vi "Main Tclk.vi"() -> ()   [LabVIEW 2018] (continued)
                        n7248 = Bundle By Name(cluster=w1400, "Low mag scan"=w1398, "Prior to main scan"=w1397, "Low mag interval"=w1396, "Low mag scan rate (Hz)"=w1395, "Show HM box"=w1394) -> (w1399:T30)
                        n7249 = local write "Low Mag SEM"(w1399) -> ()
                        n7250 = local write "Mid Mag SEM"(w1392) -> ()
                      }
                      frame #2 {
                        n7251 = Unbundle By Name(w1407) -> ("Line milling time (s)"=w1404:sgl, "Lines auto pause"=w1403:u16, "Auto Profile"=w1402:bool)
                        n7252 = local read "Milling para"() -> (w1406:T35)
                        n7253 = Bundle By Name(cluster=w1406, "Line milling time (s)"=w1404, "Lines auto pause"=w1403, "Auto Profile"=w1402) -> (w1405:T35)
                        n7254 = local write "Milling para"(w1405) -> ()
                      }
                    }
                  }
                  frame True {
                    n7255 = local write "SEM Scan Parameters"(w1427) -> ()
                    n7256 = local write "Detector Information"(w1413) -> ()
                    n7257 = local write "SEM Options"(w1426) -> ()
                    n7258 = local write "File Information"(w1425) -> ()
                    n7259 = local write "Low Mag SEM"(w1424) -> ()
                    n7260 = local write "Mid Mag SEM"(w1416) -> ()
                    n7261 = local write "FIB-SEM Angle"(w1423) -> ()
                    n7262 = local write "Milling para"(w1422) -> ()
                    n7263 = local write "X shift (nm/image)"(w1420) -> ()
                    n7264 = local write "Y shift (nm/image)"(w1421) -> ()
                    n7265 = local write "FIB Y zoom pixel (nm)"(w1419) -> ()
                    n7266 = local write "Mail server"(w1418) -> ()
                    n7267 = local write "Email Alert Recipients"(w1417) -> ()
                    n7268 = Unbundle By Name(w1413) -> ("Brightness A"=w1412:dbl, "Contrast A"=w1411:dbl, "Detector B name"=w1410:string, "Brightness B"=w1409:dbl, "Contrast B"=w1408:dbl)
                    n7269 = local read "Hardware Configuration"() -> (w1415:T25)
                    n7270 = Bundle By Name(cluster=w1415, "Brightness A"=w1412, "Contrast A"=w1411, "Detector B name"=w1410, "Brightness B"=w1409, "Contrast B"=w1408) -> (w1414:T25)
                    n7271 = local write "Hardware Configuration"(w1414) -> ()
                  }
                }
              }
              frame #1 {
                n7272 = local read "Hardware Configuration"() -> (w1448:T25)
                n7273 = local read "SEM Scan Parameters"() -> (w1432:T26)
                n7274 = local read "SEM Options"() -> (w1449:T27)
                n7275 = local read "SEM Status"() -> (w1450:T12)
                n7276 = local read "X full scale (V)"() -> (w1451:sgl)
                n7277 = local read "Mid Mag SEM"() -> (w1447:T29)
                n7278 = local read "SEM Mid Mag Scan Parameters"() -> (w1446:T5)
                n7279 = Unbundle By Name(w1447) -> ("X size (um)"=w1443:sgl, "Y size (um)"=w1442:sgl, "X center (um)"=w1441:dbl, "Y center (um)"=w1440:dbl, "Mid mag scan rate (Hz)"=w1445:u32, "Pixel size (nm)"=w1444:sgl)
                n7280 = call "SEM Scan Parameter Coerce.vi"("X full scale (V)"=w1451, "AI upper limit"=50000000.0, "SEM Status"=w1450, "SEM Options"=w1449, "SEM Scan Parameters"=w1432, "Hardware Configuration"=w1448) -> ("Coerced SEM Scan Parameters"=w1452:T5, "SEM FOV"=w1431:dbl, "Detector number"=w1430:i16)  [unwired: 3 in]
                n7281 = local write "Detector number"(w1430) -> ()
                n7282 = local write "SEM FOV"(w1431) -> ()
                n7283 = Bundle By Name(cluster=w1446, "X size (um)"=w1443, "Y size (um)"=w1442, "X center (um)"=w1441, "Y center (um)"=w1440, "Scan rate (Hz)"=w1445, "Pixel size (nm)"=w1444, "X size auto"=TRUE) -> (w1439:T5)
                n7284 = call "SEM Scan Parameter Coerce.vi"("X full scale (V)"=w1451, "SEM Status"=w1450, "SEM Options"=w1449, "SEM Scan Parameters"=w1439, "Hardware Configuration"=w1448) -> ("Coerced SEM Scan Parameters"=w1453:T5)  [unwired: 4 in, 2 out]
                n7285 = Unbundle By Name(w1453) -> ("X size (um)"=w1438:sgl, "Y size (um)"=w1437:sgl, "X center (um)"=w1436:dbl, "Y center (um)"=w1435:dbl, "Scan rate (Hz)"=w1434:u32, "Pixel size (nm)"=w1433:sgl)
                n7286 = Bundle By Name(cluster=w1447, "X size (um)"=w1438, "Y size (um)"=w1437, "X center (um)"=w1436, "Y center (um)"=w1435, "Mid mag scan rate (Hz)"=w1434, "Pixel size (nm)"=w1433) -> (w1454:T29)
                n7287 = local write "SEM Scan Parameters"(w1452) -> ()
                n7288 = local write "SEM Mid Mag Scan Parameters"(w1453) -> ()
                n7289 = local write "Mid Mag SEM"(w1454) -> ()
              }
              frame #2 {
                n7290 = local read "Milling para"() -> (w1477:T35)
                n7291 = local read "FIB"() -> (w1476:bool)
                n7292 = case shown="False" w1476 {
                  tunnel: [TRUE ("Origin") FALSE ("Origin")] -> w1475
                  tunnel: [0.0 ("Y offset pre (um)") w1480] -> w1457
                  frame False {
                  }
                  frame True {
                    n7293 = local read "Y offset pre (um)"() -> (w1480:dbl)
                  }
                }
                n7294 = Unbundle By Name(w1477) -> ("X size (um)"=w1464:sgl, "Z size (um)"=w1465:sgl, "Z-step (nm)"=w1455:dbl)
                n7295 = expression code="x/1e3"(w1455) -> (w1467:dbl)
                n7296 = control-ref of="FIB Image"() -> (w1471:refnum<vi>)
                n7297 = local read "FIB Scan Parameters"() -> (w1472:T32)
                n7298 = local read "FIB Options"() -> (w1473:T33)
                n7299 = shared-variable ".\\Zeiss Library.lvlib\\Milling Z Voltage RT"() -> (w1474:sgl)  [unwired: 1 in, 1 out]
                n7300 = expression code="log2( x/0.1)"(w1464) -> (w1462:sgl)
                n7301 = Round Toward +Infinity(x=w1462) -> (ceil(x): smallest int >= x=w1460:sgl)
                n7302 = call "FIB image draw milling.vi"("Milling Z Voltage"=w1474, "Milling para"=w1477, "Z offset pre (um)"=w1457, "FIB Options"=w1473, "FIB Scan Parameters"=w1472, "Origin"=w1475, "Image reference"=w1471) -> ("Trapezoidal"=w1456:cluster{"X":i16, "Y":i16}[])  [unwired: 3 in, 1 out]
                n7303 = Scale By Power Of 2(n=w1460, x=ext 1.0) -> (x*2^n=w1463:ext)
                n7304 = local write "Trapezoidal"(w1456) -> ()
                n7305 = Divide(x=w1465, y=w1467) -> (x/y=w1459:dbl)
                n7306 = Round To Nearest(number=w1459) -> (nearest integer value=w1470:dbl)
                n7307 = local read "Milling para"() -> (w1468:T35)
                n7308 = Increment(x=w1470) -> (x+1=w1469:dbl)
                n7309 = Multiply(x=w1470, y=w1467) -> (x*y=w1466:dbl)
                n7310 = Bundle By Name(cluster=w1468, "X resolution"=w1463, "Z resolution"=w1469, "Z size (um)"=w1466) -> (w1458:T35)
                n7311 = local write "Milling para"(w1458) -> ()
              }
              frame #3 {
                n7312 = local read "dat to csv and xml"() -> (w1482:bool)
                n7313 = local write "Load recipe"(FALSE ("Load recipe")) -> ()
                n7314 = case shown="True" w1482 {
                  frame False {
                  }
                  frame True {
                    n7315 = stacked-sequence {
                      frame #0 {
                        w1484 = u32 10 ("Remaining X shift frames")
                        w1500 = i16 60 ("top")
                        n7316 = local read "SEM Scan Parameters"() -> (w1495:T26)
                        n7317 = local read "Recipe input"() -> (w1527:T7)
                        n7318 = local read "Last FIB recipe"() -> (w1528:path)
                        n7319 = local read "Read recipe path"() -> (w1514:path)
                        n7320 = Path To String(path=w1514) -> (string=w1513:string)
                        n7321 = call "Recipe read write.vi"("Write"=TRUE, "Recipe path"=w1528, "Write input"=w1527) -> ()  [unwired: 5 in, 4 out]
                        n7322 = call "Zeiss File Header Tclk.vi"("Write"=FALSE, "Input file path"=w1514) -> ("Ouputs"=w1522:T79)  [unwired: 7 in, 2 out]
                        n7323 = Unbundle By Name(w1495) -> ("X size (um)"=w1494:sgl, "Y size (um)"=w1491:sgl, "Pixel size (nm)"=w1493:sgl)
                        n7324 = local read "Hardware Configuration"() -> (w1487:T25)
                        n7325 = Unbundle By Name(w1522) -> ("Data Logging.Milling Z voltage (V)"=w1520:sgl, "Data Logging.FIB slice #"=w1518:u32, "Data Logging.Focus Index"=w1517:sgl, "Decimating factor"=w1488:u16)
                        n7326 = call "Timestamp from dat file.vi"("dat file path"=w1514) -> ("time stamp"=w1519:timestamp)  [unwired: 10 in]
                        n7327 = Search and Replace String(input string=w1513, search string=".dat", replace string=".png" ("replace string (\"\")")) -> (result string=w1510:string)  [unwired: 5 in, 3 out]
                        n7328 = String To Path(string=w1510) -> (path=w1509:path)
                        n7329 = local read "Last milling snapshot"() -> (w1523:path)
                        n7330 = expression code="x/1000"(w1493) -> (w1492:sgl)
                        n7331 = Divide(x=w1494, y=w1492) -> (x/y=w1490:sgl)
                        n7332 = Divide(x=w1491, y=w1492) -> (x/y=w1489:sgl)
                        n7333 = Unbundle By Name(w1487) -> ("SEM Max FOV (um)"=w1486:sgl)
                        n7334 = Divide(x=w1490, y=w1488) -> (x/y=w1502:sgl)
                        n7335 = Divide(x=w1489, y=w1488) -> (x/y=w1499:sgl)
                        n7336 = To Word Integer(number=w1502) -> (16bit integer=w1498:i16)
                        n7337 = To Word Integer(number=w1499) -> (16bit integer=w1497:i16)
                        n7338 = local read "Re-engage Files"() -> (w1504:path)
                        n7339 = call <vilib>:"Read PNG File.vi"("path to PNG file"=w1509) -> ("image data"=w1496:T52)  [unwired: 8 in, 2 out]
                        n7340 = Add(x=w1500, y=w1497) -> (x+y=w1501:i16)
                        n7341 = Bundle(cluster=T46 {"Timestamp"=timestamp(0 s since 1904-01-01), "Milling Z voltage"=0.0, "FIB slice #"=0, "Pause for reheat"=FALSE, "Last good FI"=0.0, "Focus index"=0.0, "SEM max FOV"=0.0, "Remaining X shift frames"=0, "Remaining Y shift frames"=0} ("output cluster"), "Timestamp"=w1519, "Milling Z voltage"=w1520, "FIB slice #"=w1518, "Pause for reheat"=TRUE ("Reheat"), "Last good FI"=w1517, "Focus index"=w1517, "SEM max FOV"=w1486, "Remaining X shift frames"=w1484, "Remaining Y shift frames"=w1484) -> (w1524:T46)
                        n7342 = Bundle By Name(cluster=T47 {"left"=0, "top"=0, "right"=0, "bottom"=0} ("subset rect"), "left"=i16 0, "top"=w1500, "right"=w1498, "bottom"=w1501) -> (w1506:T47)
                        n7343 = Flatten To XML(anything=w1524) -> (xml string=w1525:string)
                        n7344 = call-poly <vilib>:"Write to XML File.vi"("XML Input"=w1525, "XML File Path"=w1523) -> ()  [unwired: 7 in, 3 out]
                        n7345 = call <vilib>:"Get Image Subset.vi"("subset rect"=w1506, "image data"=w1496) -> ("image subset"=w1515:T52)  [unwired: 4 in, 1 out]
                        n7346 = Build Path(base path=w1504, name or relative path="pre.png") -> (appended path=w1503:path)
                        n7347 = call <vilib>:"Write PNG File.vi"("image data"=w1515, "path to PNG file"=w1503) -> ()  [unwired: 1 in, 9 out]
                      }
                      frame #1 {
                        n7348 = local write "dat to csv and xml"(FALSE ("dat to csv and xml")) -> ()
                        n7349 = local read "Milling para"() -> (w1529:T35)
                        n7350 = Bundle By Name(cluster=w1529, "Mill start from Last"=TRUE) -> (w1531:T35)
                        n7351 = local write "Milling para"(w1531) -> ()
                      }
                    }
                  }
                }
              }
            }
          }
        }
        n7352 = local read "Stop"() -> (w1329:bool)
      }
      n7353 = while {
        shift-right: [w1616] -> _
        shift-left: w707 -> [w1615]
        shift-right: [w1611] -> _
        shift-left: _ -> [w1612]
        shift-right: [w1606] -> _
        shift-left: w707 -> [w1605]
        shift-right: [w1604] -> _
        shift-left: w707 -> [w1594]
        shift-right: [w1597] -> _
        shift-left: w707 -> [w1596]
        shift-right: [w1589] -> _
        shift-left: w707 -> [w1588]
        shift-right: ["Start FIB HV DataLog"] -> _
        shift-left: _ -> [w1587]
        shift-right: [w1583] -> _
        shift-left: w707 -> [w1578]
        shift-right: [w1574] -> _
        shift-left: w707 -> [w1567]
        stop <- w1613 stop-if-true
        n7354 = local read "FIB"() -> (w1599:bool)
        n7355 = local read "FIB slice #"() -> (w1593:u32)
        n7356 = local read "Mill Manual Pause"() -> (w1591:bool)
        n7357 = local read "SW error warning armed"() -> (w1575:bool)
        n7358 = local read "Alert Settings"() -> (w1554:T36)
        n7359 = local read "Milling para"() -> (w1552:T35)
        n7360 = Tick Count (ms)() -> (millisecond timer value=w1611:u32)
        n7361 = Equal To 0?(x=w1594) -> (x = 0?=w1600:bool)
        n7362 = local read "Machine Type"() -> (w1576:u8)
        n7363 = Equal To 0?(x=w1578) -> (x = 0?=w1577:bool)
        n7364 = Equal To 0?(x=w1567) -> (x = 0?=w1566:bool)
        n7365 = Subtract(x=w1611, y=w1612) -> (x-y=w1570:u32)
        n7366 = Not Equal?(x=w1587, y="Start FIB HV DataLog") -> (x != y?=w1586:bool)
        n7367 = Equal To 0?(x=w1605) -> (x = 0?=w1537:bool)
        n7368 = Not Equal To 0?(x=w1593) -> (x != 0?=w1592:bool)
        n7369 = And(x=w1586, y="Start FIB HV DataLog") -> (x .and. y?=w1585:bool)
        n7370 = Unbundle By Name(w1552) -> ("Lines auto pause"=w1551:u16)
        n7371 = Wait Until Next ms Multiple(millisecond multiple=u32 1000) -> ()  [unwired: 1 out]
        n7372 = Unbundle By Name(w1554) -> ("SW error warning"=w1553:bool)
        n7373 = Compound Arithmetic op=AND(w1566, "Start Current DataLog") -> (w1564:bool)
        n7374 = Not(x=w1591) -> (.not. x?=w1590:bool)
        n7375 = case shown="True" w1537 {
          frame False {
          }
          frame True {
            w1845 = 10.0 ("y")
            w1851 = 50 ("sample length")
            n7376 = local read "Hardware Configuration"() -> (w1837:T25)
            n7377 = for {
              N: w1851 -> [_]
              tunnel: [w1862] -> w1850 mode=indexing
              i -> [w1862]
            }
            n7378 = Unbundle By Name(w1837) -> ("Temperature port"=w1838:refnum<visa-resource-name>)
            n7379 = for {
              N: 3 -> [_]
              tunnel: w1838 -> [w1860]
              tunnel: [w1857] -> w1855
              stop <- w1858 stop-if-true
              w1861 = TRUE ("Close session")
              n7380 = call "Watchport Comm.vi"("Close session"=w1861, "Initialization"=w1861, "Watchport command"="TF", "Watchport COM #"=w1860) -> ("value"=w1857:sgl)  [unwired: 3 in, 4 out]
              n7381 = Not Equal To 0?(x=w1857) -> (x != 0?=w1858:bool)
              n7382 = Wait Until Next ms Multiple(millisecond multiple=u32 100) -> ()  [unwired: 1 out]
            }
            "Temp (F)" <- w1855
            n7383 = call <vilib>:"Data Queue PtByPt.vi"("sample length"=w1851, "input data point"=w1855) -> ("Current Queue"=w1852:dbl[])  [unwired: 5 in, 4 out]
            n7384 = call "Remove value from array.vi"("Value to remove"=0.0, "Input array"=w1852) -> ("Output array"=w1842:dbl[])  [unwired: 8 in, 1 out]
            n7385 = Array Size(array=w1842) -> (size(s)=w1843:i32)
            n7386 = Array Subset(array=w1850, length=w1843) -> (w1849:i32[])  [unwired: 1 in]
            n7387 = call <vilib>:"Linear Fit.vi"("Y"=w1842, "X"=w1849) -> ("slope"=w1854:dbl)  [unwired: 9 in, 4 out]
            n7388 = Multiply(x=w1854, y=w1845) -> (x*y=w1848:dbl)
            n7389 = Less Or Equal?(x=w1845, y=w1843) -> (x <= y?=w1844:bool)
            n7390 = Select(t=w1848, s=w1844, f=0.0) -> (s? t:f=→"Temp gradient (F/min)":dbl)
            n7391 = Array Max & Min(array=w1842) -> (max value=w1841:dbl, min value=w1840:dbl)  [unwired: 2 out]
            n7392 = Subtract(x=w1841, y=w1840) -> (x-y=→"Temp range (F)":dbl)
          }
        }
        n7393 = Add(x=w1570, y=w1594) -> (x+y=w1603:u32)
        n7394 = case shown="True" "Start FIB HV DataLog" {
          tunnel: [u32 0 ("f") w1687] -> w1589
          tunnel: w1570 -> [_ w1686]
          tunnel: w1588 -> [_ w1685]
          tunnel: w1585 -> [_ w1684]
          tunnel: w1576 -> [_ w1683]
          frame False {
          }
          frame True {
            n7395 = case shown="0" w1683 {
              tunnel: [w1696 u32 0 ("f") w1764] -> w1687
              tunnel: w1686 -> [w1695 _ w1763]
              tunnel: w1685 -> [w1694 _ w1762]
              tunnel: w1684 -> [w1691 _ w1758]
              frame 0 {
                n7396 = Equal To 0?(x=w1694) -> (x = 0?=w1689:bool)
                n7397 = local read "Re-read HVDataLog"() -> (w1690:bool)
                n7398 = Or(x=w1689, y=w1690) -> (x .or. y?=w1688:bool)
                n7399 = case shown="True" w1688 {
                  tunnel: w1691 -> [_ w1700]
                  frame False {
                  }
                  frame True {
                    n7400 = stacked-sequence {
                      tunnel: w1700 -> [w1701 _]
                      frame #0 {
                        n7401 = local read "FIB HV DataLog Files"() -> (w1702:path)
                        n7402 = Get Date/Time In Seconds() -> (seconds since 1Jan1904=w1709:timestamp)
                        n7403 = case shown="True" w1701 {
                          frame False {
                          }
                          frame True {
                            w1711 = 0.0
                            n7404 = Get Date/Time In Seconds() -> (seconds since 1Jan1904=w1721:timestamp)
                            n7405 = To Double Precision Float(number=w1721) -> (double precision float=w1716:dbl)
                            n7406 = Bundle(w1711, w1711) -> (w1710:cluster{dbl, dbl})  [unwired: 1 in]
                            n7407 = Add(x=w1716, y=86400.0 ("X Scale.Range:Maximum")) -> (x+y=w1718:dbl)
                            n7408 = Initialize Array(w1710, 0) -> (w1713:cluster{dbl, dbl}[])
                            n7409 = Add(x=w1716, y=0.0 ("X Scale.Range:Minimum")) -> (x+y=w1714:dbl)
                            n7410 = property on="FIB HV DataLog" class="WFChart (strict)"("History Data"=w1713, "XScale.Offset"=w1716, "XScale.Minimum"=w1714, "XScale.Maximum"=w1718, "XScale.Increment"=14400.0 ("X Scale.Range:Increment"), "XScale.MinorInc"=3600.0 ("X Scale.Range:Minor Increment")) -> ()  [unwired: 2 in, 2 out]
                          }
                        }
                        n7411 = Format Date/Time String(time format string (%c)="Y%Y\\M%m\\D%d", seconds (now)=w1709) -> (date/time string=w1705:string)  [unwired: 1 out]
                        n7412 = Build Path(base path=w1702, name or relative path=w1705) -> (appended path=w1703:path)
                        n7413 = File/Directory Info(path=w1703) -> (path out=w1708:path, error out=w1706:errorcluster)  [unwired: 1 in, 5 out]
                        n7414 = Unbundle By Name(w1706) -> ("status"=w1707:bool)
                        n7415 = case shown="True" w1707 {
                          tunnel: w1708 -> [_ w1722]
                          frame False {
                          }
                          frame True {
                            n7416 = Create Folder(path (use dialog)=w1722) -> ()  [unwired: 1 in, 4 out]
                          }
                        }
                      }
                      frame #1 {
                        n7417 = call "Read FIB Log Files.vi"("Log file path"=path "C:/Program Files (x86)/FEI Company/BDS/LogHVData.log") -> ("HV Data Output"=w1729:T118)  [unwired: 9 in, 1 out]
                        n7418 = Unbundle By Name(w1729) -> ("Filament (A)"=w1745:sgl, "Acclerator (V)"=w1744:sgl, "AccI (uA)"=w1743:sgl, "Extractor (V)"=w1742:sgl, "Emission (uA)"=w1730:sgl, "Suppressor (V)"=w1731:sgl, "SuppI (uA)"=w1741:sgl, "Lens1 (V)"=w1740:sgl, "Lens1I (uA)"=w1739:sgl, "Lens2 (V)"=w1738:sgl, "Lens2I (uA)"=w1737:sgl, "Tip Lifetime (hr)"=w1728:sgl)
                        n7419 = local read "Faraday Cup RT"() -> (w1726:sgl)
                        n7420 = local read "Specimen RT"() -> (w1725:sgl)
                        n7421 = local read "BD1 RT"() -> (w1724:sgl)
                        n7422 = local read "BD2 RT"() -> (w1723:sgl)
                        n7423 = Build Array(w1745, w1744, w1743, w1742, w1730, w1731, w1741, w1740, w1739, w1738, w1737, w1728, w1726, w1725, w1724, w1723) -> (w1733:sgl[])
                        n7424 = Bundle("Suppressor (V)"=w1731, "Emission (uA)"=w1730) -> (w1732:T122)  [unwired: 1 in]
                        n7425 = Add Array Elements(numeric array=w1733) -> (sum=w1734:sgl)
                        n7426 = Equal To 0?(x=w1734) -> (x = 0?=w1736:bool)
                        n7427 = Equal To 0?(x=w1728) -> (x = 0?=w1735:bool)
                        n7428 = And(x=w1736, y=w1735) -> (x .and. y?=w1727:bool)
                        "Re-read HVDataLog" <- w1727
                        n7429 = case shown="False" w1727 {
                          tunnel: w1733 -> [w1750 _]
                          tunnel: w1732 -> [w1754 _]
                          tunnel: w1729 -> [w1747 _]
                          frame False {
                            n7430 = local read "FIB HV DataLog Files"() -> (w1752:path)
                            n7431 = Get Date/Time In Seconds() -> (seconds since 1Jan1904=w1751:timestamp)
                            n7432 = for {
                              tunnel: w1750 -> [w1756] mode=indexing
                              tunnel: [w1755] -> w1749 mode=indexing
                              n7433 = Format Into String(w1756) -> (resulting string=w1755:string)  [unwired: 3 in, 1 out]
                            }
                            n7434 = call "YMD log files.vi"("Input text array"=w1749, "Input header array"=string[] ["Date", "Time", "Filament Current (A)", "Accelerator (V)", "Accelerator I (uA)", "Extractor (V)", "Emission (uA)", "Suppressor (V)", "Suppressor I (uA)", "Lens 1 (V)", "Lens 1 I (uA)", "Lens 2 (V)", "Lens 2 I (uA)", "Tip Lifetime (hr)", "Faraday Cup (nA)", "Specimen (nA)", "Beam Dump 1 (nA)", "Beam Dump 2 (nA)"], "current time"=w1751, "Log file name"="HVDataLog" ("string"), "Log file path"=w1752) -> ()  [unwired: 7 in]
                            "FIB HV DataLog" <- w1754
                            "HV Data Output" <- w1747
                          }
                          frame True {
                          }
                        }
                      }
                    }
                  }
                }
                n7435 = Add(x=w1695, y=w1694) -> (x+y=w1698:u32)
                n7436 = expression code="x*1000"("Interval (s)") -> (w1693:u16)
                n7437 = Less?(x=w1698, y=w1693) -> (x < y?=w1699:bool)
                n7438 = Select(t=w1698, s=w1699, f=u32 0) -> (s? t:f=w1696:u32)
                n7439 = property on="FIB HV DataLog" class="WFChart (strict)"("XScale.Multiplier"="Interval (s)") -> ()  [unwired: 2 in, 2 out]
              }
              frame 1, Default {
              }
              frame 2 {
                n7440 = Equal To 0?(x=w1762) -> (x = 0?=w1765:bool)
                n7441 = local read "Re-read HVDataLog"() -> (w1766:bool)
                n7442 = Or(x=w1765, y=w1766) -> (x .or. y?=w1759:bool)
                n7443 = case shown="True" w1759 {
                  tunnel: w1758 -> [_ w1770]
                  frame False {
                  }
                  frame True {
                    n7444 = stacked-sequence {
                      tunnel: w1770 -> [w1774 _]
                      frame #0 {
                        n7445 = local read "FIB HV DataLog Files"() -> (w1775:path)
                        n7446 = local read "Api"() -> (w1771:refnum<k7>)
                        n7447 = call "SmartSEM Remote API get FIB HV data.vi"("ActiveX Container"=w1771) -> ("error out"=w1773:errorcluster, "Capella HV Data Output"=w1772:T17)  [unwired: 7 in, 2 out]
                        n7448 = Get Date/Time In Seconds() -> (seconds since 1Jan1904=w1782:timestamp)
                        n7449 = local write "Capella HV Data Output"(w1772) -> ()
                        n7450 = Format Date/Time String(time format string (%c)="Y%Y\\M%m\\D%d", seconds (now)=w1782) -> (date/time string=w1778:string)  [unwired: 1 out]
                        n7451 = Build Path(base path=w1775, name or relative path=w1778) -> (appended path=w1776:path)
                        n7452 = File/Directory Info(path=w1776) -> (path out=w1781:path, error out=w1779:errorcluster)  [unwired: 1 in, 5 out]
                        n7453 = case shown="True" w1774 {
                          tunnel: w1773 -> [_ _]
                          frame False {
                          }
                          frame True {
                            w1784 = 0.0
                            n7454 = Get Date/Time In Seconds() -> (seconds since 1Jan1904=w1794:timestamp)
                            n7455 = To Double Precision Float(number=w1794) -> (double precision float=w1789:dbl)
                            n7456 = Bundle(w1784, w1784) -> (w1783:cluster{dbl, dbl})  [unwired: 1 in]
                            n7457 = Add(x=w1789, y=86400.0 ("X Scale.Range:Maximum")) -> (x+y=w1791:dbl)
                            n7458 = Initialize Array(w1783, 0) -> (w1786:cluster{dbl, dbl}[])
                            n7459 = Add(x=w1789, y=0.0 ("X Scale.Range:Minimum")) -> (x+y=w1787:dbl)
                            n7460 = property on="FIB HV DataLog" class="WFChart (strict)"("History Data"=w1786, "XScale.Offset"=w1789, "XScale.Minimum"=w1787, "XScale.Maximum"=w1791, "XScale.Increment"=14400.0 ("X Scale.Range:Increment"), "XScale.MinorInc"=3600.0 ("X Scale.Range:Minor Increment")) -> ()  [unwired: 2 in, 2 out]
                          }
                        }
                        n7461 = Unbundle By Name(w1779) -> ("status"=w1780:bool)
                        n7462 = case shown="True" w1780 {
                          tunnel: w1781 -> [_ w1795]
                          frame False {
                          }
                          frame True {
                            n7463 = Create Folder(path (use dialog)=w1795) -> ()  [unwired: 1 in, 4 out]
                          }
                        }
                      }
                      frame #1 {
                        n7464 = local read "Capella HV Data Output"() -> (w1796:T17)
                        n7465 = Unbundle By Name(w1796) -> ("Filament (A)"=w1817:sgl, "Accelerator Target (V)"=w1816:sgl, "Accelerator Actual (V)"=w1815:sgl, "Extrator Target (V)"=w1814:sgl, "Extrator Actual (V)"=w1813:sgl, "Emission Target (uA)"=w1812:sgl, "Emission Actual (uA)"=w1805:sgl, "Suppressor (V)"=w1806:sgl, "Lens1 Target (V)"=w1811:sgl, "Lens1 Actual (V)"=w1810:sgl, "Lens2 Target (V)"=w1809:sgl, "Lens2 Actual (V)"=w1808:sgl, "Tip Lifetime (uAhr)"=w1804:sgl, "Gun Vac (Torr)"=w1803:sgl, "Column Vac (Torr)"=w1802:sgl)
                        n7466 = Bundle("Suppressor (V)"=w1806, "Emission Actual (uA)"=w1805) -> (w1818:T123)  [unwired: 1 in]
                        n7467 = Build Array(w1817, w1816, w1815, w1814, w1813, w1812, w1805, w1806, w1811, w1810, w1809, w1808, w1804) -> (w1807:sgl[])
                        n7468 = Build Array(w1803, w1802) -> (w1801:sgl[])
                        n7469 = local write "FIB HV DataLog"(w1818) -> ()
                        n7470 = for {
                          tunnel: w1807 -> [w1827] mode=indexing
                          tunnel: [w1826] -> w1799 mode=indexing
                          n7471 = Format Into String(w1827) -> (resulting string=w1826:string)  [unwired: 3 in, 1 out]
                        }
                        n7472 = for {
                          tunnel: w1801 -> [w1825] mode=indexing
                          tunnel: [w1824] -> w1798 mode=indexing
                          tunnel: "%e" ("format string") -> [w1823]
                          n7473 = Format Into String(format string=w1823, w1825) -> (resulting string=w1824:string)  [unwired: 2 in, 1 out]
                        }
                        n7474 = Build Array (concatenate)(w1799, w1798) -> (w1797:string[])
                        n7475 = local read "FIB HV DataLog Files"() -> (w1821:path)
                        n7476 = Get Date/Time In Seconds() -> (seconds since 1Jan1904=w1820:timestamp)
                        n7477 = call "YMD log files.vi"("Input text array"=w1797, "Input header array"=string[] ["Date", "Time", "Filament Current (A)", "Accelerator Target (V)", "Accelerator Actual (V)", "Extractor Target (V)", "Extractor Actual (V)", "Emission Target (uA)", "Emission Actual (uA)", "Suppressor (V)", "Lens 1 Target (V)", "Lens 1 Actual (V)", "Lens 2 Target (V)", "Lens 2 Actual (uA)", "Tip Lifetime (hr)", "Gun Vacuum (Torr)", "Column Vacuum (Torr)", ""], "current time"=w1820, "Log file name"="HVDataLog" ("string"), "Log file path"=w1821) -> ()  [unwired: 7 in]
                      }
                    }
                  }
                }
                n7478 = local read "Interval (s)"() -> (w1761:u16)
                n7479 = Add(x=w1763, y=w1762) -> (x+y=w1760:u32)
                n7480 = expression code="x*1000"(w1761) -> (w1767:u16)
                n7481 = Less?(x=w1760, y=w1767) -> (x < y?=w1769:bool)
                n7482 = Select(t=w1760, s=w1769, f=u32 0) -> (s? t:f=w1764:u32)
                n7483 = property on="FIB HV DataLog" class="WFChart (strict)"("XScale.Multiplier"=w1761) -> ()  [unwired: 2 in, 2 out]
              }
            }
          }
        }
        n7484 = case shown="2" w1576 {
          frame 0, Default {
          }
          frame 2 {
            n7485 = local read "Status message"() -> (w1643:string)
            n7486 = Equal?(x=w1643, y="SEM between FIB" ("Status message")) -> (x = y?=w1641:bool)
            n7487 = case shown="False" w1641 {
              frame False {
                n7488 = local read "Api"() -> (w1646:refnum<k7>)
                n7489 = call "SmartSEM Remote API FIB gun state.vi"("ActiveX Container"=w1646) -> ("error out"=w1644:errorcluster, "FIB Gun State"=w1650:string)  [unwired: 8 in, 1 out]
                "FIB Gun State" <- w1650
                n7490 = case shown="\"Regulating\"" w1650 {
                  tunnel: w1646 -> [_ _ _ _ _ _ _ _ _ _ _ _ _ _ w1673 _ _ _ _ _ _]
                  tunnel: w1644 -> [_ _ _ _ _ _ _ _ _ _ _ _ _ _ w1669 _ _ _ _ _ _]
                  frame "Off", Default {
                    n7491 = property on="Turn off FIB gun" class="Bool (strict)"("DisabledEnum"=T44."Disabled and Grayed Out" ("Disabled")) -> ()  [unwired: 2 in, 2 out]
                    n7492 = property on="Turn on FIB gun" class="Bool (strict)"("DisabledEnum"=T44."Enabled" ("Disabled")) -> ()  [unwired: 2 in, 2 out]
                    n7493 = local write "Turn off FIB gun"(TRUE ("Turn on FIB gun")) -> ()
                    n7494 = local write "Turn on FIB gun"(FALSE ("Turn on FIB gun")) -> ()
                  }
                  frame "On" {
                    w1657 = FALSE ("Turn on FIB gun")
                    w1658 = T44."Enabled" ("Disabled")
                    n7495 = property on="Turn on FIB gun" class="Bool (strict)"("DisabledEnum"=T44."Disabled and Grayed Out" ("Disabled")) -> ()  [unwired: 2 in, 2 out]
                    n7496 = property on="Turn off FIB gun" class="Bool (strict)"("DisabledEnum"=w1658) -> ()  [unwired: 2 in, 2 out]
                    n7497 = property on="Turn FIB gun standby" class="Bool (strict)"("DisabledEnum"=w1658) -> ()  [unwired: 2 in, 2 out]
                    n7498 = local write "Turn on FIB gun"(TRUE ("Turn on FIB gun")) -> ()
                    n7499 = local write "Turn FIB gun standby"(w1657) -> ()
                    n7500 = local write "Turn off FIB gun"(w1657) -> ()
                  }
                  frame "Ramping" {
                  }
                  frame "Error" {
                  }
                  frame "Vac Not Ready" {
                  }
                  frame "Extractor Auto" {
                  }
                  frame "Heating" {
                  }
                  frame "Conditioning" {
                  }
                  frame "Filament Heating" {
                  }
                  frame "Gun colling down" {
                  }
                  frame "Ramping Down" {
                  }
                  frame "Standby" {
                    w1662 = FALSE ("Turn on FIB gun")
                    w1661 = T44."Enabled" ("Disabled")
                    n7501 = property on="Turn on FIB gun" class="Bool (strict)"("DisabledEnum"=w1661) -> ()  [unwired: 2 in, 2 out]
                    n7502 = property on="Turn off FIB gun" class="Bool (strict)"("DisabledEnum"=w1661) -> ()  [unwired: 2 in, 2 out]
                    n7503 = property on="Turn FIB gun standby" class="Bool (strict)"("DisabledEnum"=T44."Disabled and Grayed Out" ("Disabled")) -> ()  [unwired: 2 in, 2 out]
                    n7504 = local write "Turn on FIB gun"(w1662) -> ()
                    n7505 = local write "Turn off FIB gun"(w1662) -> ()
                    n7506 = local write "Turn FIB gun standby"(TRUE ("Turn on FIB gun")) -> ()
                  }
                  frame "FIB Emission Failed" {
                    n7507 = property on="Turn off FIB gun" class="Bool (strict)"("DisabledEnum"=T44."Enabled" ("Disabled")) -> ()  [unwired: 2 in, 2 out]
                    n7508 = property on="Turn on FIB gun" class="Bool (strict)"("DisabledEnum"=T44."Enabled" ("Disabled")) -> ()  [unwired: 2 in, 2 out]
                    n7509 = local write "Turn on FIB gun"(FALSE ("Turn on FIB gun")) -> ()
                    n7510 = local write "Turn off FIB gun"(FALSE ("Turn on FIB gun")) -> ()
                  }
                  frame "Going to regulating" {
                  }
                  frame "Regulating" {
                    w1670 = TRUE ("Turn on FIB gun")
                    w1676 = FALSE ("Turn on FIB gun")
                    w1677 = T44."Enabled" ("Disabled")
                    n7511 = call "SmartSEM Remote API get FIB HV data.vi"("error in"=w1669, "ActiveX Container"=w1673) -> ("Capella HV Data Output"=w1671:T17)  [unwired: 6 in, 3 out]
                    "Capella HV Data Output" <- w1671
                    n7512 = property on="Turn on FIB gun" class="Bool (strict)"("DisabledEnum"=T44."Disabled and Grayed Out" ("Disabled")) -> ()  [unwired: 2 in, 2 out]
                    n7513 = property on="Turn off FIB gun" class="Bool (strict)"("DisabledEnum"=w1677) -> ()  [unwired: 2 in, 2 out]
                    n7514 = property on="Turn FIB gun standby" class="Bool (strict)"("DisabledEnum"=w1677) -> ()  [unwired: 2 in, 2 out]
                    n7515 = call "FIB HV target match.vi"("Capella HV Data Output"=w1671) -> ("Max absolute error (V)"=w1674:sgl)  [unwired: 5 in, 5 out]
                    n7516 = Less?(x=w1674, y=sgl 80.0) -> (x < y?=→"FIB HV target matched":bool)
                    n7517 = local write "Turn on FIB gun"(w1670) -> ()
                    n7518 = local write "Start FIB HV DataLog"(w1670) -> ()
                    n7519 = local write "Turn off FIB gun"(w1676) -> ()
                    n7520 = local write "Turn FIB gun standby"(w1676) -> ()
                  }
                  frame "Going to Standby" {
                  }
                  frame "Multi-Heating (Heater is ON)" {
                  }
                  frame "Emission Recovery (Heater is OFF)" {
                  }
                  frame "No User Has Logged On" {
                    n7521 = local write "Status message"("No user has logged on to SmartSEM" ("Status message")) -> ()
                  }
                  frame "No user is logged on" {
                    n7522 = local write "Status message"("No user is logged on to SmartSEM" ("Status message")) -> ()
                  }
                  frame "API not initialized" {
                    n7523 = local write "Status message"("API not initialized" ("Status message")) -> ()
                  }
                }
                n7524 = call "SmartSEM Remote API get string.vi"("error in"=w1644, "lpszParam"="DP_FIB_GUN_VALVE", "ActiveX Container"=w1646) -> ("data"=w1645:string)  [unwired: 6 in, 2 out]
                n7525 = Concatenate Strings("FIB Gun Valve is " ("lpszCommand"), w1645) -> (→"FIB Gun Valve Status":string)
                n7526 = case shown="\"Closed\", Default" w1645 {
                  frame "Open" {
                    n7527 = local write "Open FIB gun valve"(TRUE ("Open FIB gun valve")) -> ()
                  }
                  frame "Closed", Default {
                    n7528 = local write "Open FIB gun valve"(FALSE ("Open FIB gun valve")) -> ()
                  }
                }
              }
              frame True {
              }
            }
          }
        }
        n7529 = case shown="True" w1577 {
          tunnel: w1576 -> [_ w1635]
          frame False {
          }
          frame True {
            n7530 = case shown="2" w1635 {
              frame 0, Default {
              }
              frame 2 {
                n7531 = local read "Api"() -> (w1640:refnum<k7>)
                n7532 = local read "SEM HV DataLog Files"() -> (w1639:path)
                n7533 = call "SEM HV log.vi"("SEM HV DataLog Files Directory"=w1639, "ActiveX Container"=w1640) -> ("error out"=w1637:errorcluster, "SEM HV Data Output"=→"SEM HV Data Output":T16)  [unwired: 7 in, 1 out]
                n7534 = Unbundle By Name(w1637) -> ("status"=w1636:bool)
                n7535 = local write "API timeout"(w1636) -> ()
              }
            }
          }
        }
        n7536 = case shown="True" w1564 {
          frame False {
          }
          frame True {
            n7537 = local read "COM port"() -> (w1631:refnum<visa-resource-name>)
            n7538 = local read "Machine Type"() -> (w1632:u8)
            n7539 = local read "Api"() -> (w1633:refnum<k7>)
            n7540 = local read "Current DataLog Files"() -> (w1634:path)
            n7541 = local read "Parameter Names"() -> (w1630:string[])
            n7542 = call "Data log.vi"("COM port"=w1631, "Parameter Names"=w1630, "Machine Type"=w1632, "DataLog Files Directory"=w1634, "ActiveX Container"=w1633) -> ()  [unwired: 5 in, 2 out]
          }
        }
        n7543 = local read "Median cycle time est offset (s)"() -> (w1560:i16)
        n7544 = local read "Cycle time array"() -> (w1563:u32[])
        n7545 = Less?(x=w1551, y=u16 10) -> (x < y?=w1549:bool)
        n7546 = Compound Arithmetic op=AND(w1600, w1599, w1592, w1590, w1575, w1553, w1549) -> (w1598:bool)
        n7547 = Array Size(array=w1563) -> (size(s)=w1562:i32)
        n7548 = case shown="False" w1598 {
          tunnel: [w1828 w1831] -> w1597
          tunnel: w1596 -> [w1828 w1830]
          frame False {
          }
          frame True {
            n7549 = local read "FIB slice #"() -> (w1831:u32)
            n7550 = Equal?(x=w1831, y=w1830) -> (x = y?=w1829:bool)
            "SW error warning active" <- w1829
            n7551 = case shown="True" w1829 {
              frame False {
              }
              frame True {
                n7552 = local read "FIB HW Config"() -> (w1835:T23)
                n7553 = Unbundle By Name(w1835) -> ("Beam blank"=w1834:tag)
                n7554 = local read "Api"() -> (w1832:refnum<k7>)
                n7555 = call "FIB beam blank.vi"("ActiveX Container"=w1832, "Beam blanked"=TRUE, "lines"=w1834) -> ()  [unwired: 2 in, 1 out]
              }
            }
          }
        }
        n7556 = Greater Or Equal?(x=w1562, y=100) -> (x >= y?=w1546:bool)
        n7557 = Select(t=w1560, s=w1546, f=u32 0) -> (s? t:f=w1557:u32)
        n7558 = local read "Est. cycle time (s)"() -> (w1555:u32)
        n7559 = local read "LM overhead"() -> (w1539:u32)
        n7560 = local read "MM overhead"() -> (w1538:u32)
        n7561 = Compound Arithmetic op=ADD(u32 20 ("value"), w1557, w1555, w1539, w1538) -> (w1558:u32)
        "Timeout threshold (s)" <- w1558
        n7562 = expression code="x*1000"(w1558) -> (w1595:u32)
        n7563 = local read "FIB"() -> (w1536:bool)
        n7564 = Less?(x=w1603, y=w1595) -> (x < y?=w1602:bool)
        n7565 = case shown="True" w1536 {
          frame False {
          }
          frame True {
            n7566 = local read "Api"() -> (w1623:refnum<k7>)
            n7567 = call "SmartSEM Remote API get string.vi"("lpszParam"="DP_FIB_IMAGE_PROBE", "ActiveX Container"=w1623) -> ("data"=w1621:string, "reference out"=w1619:refnum<k7>)  [unwired: 7 in, 1 out]
            n7568 = local write "FIB Milling Probe"(w1621) -> ()
            n7569 = call "SmartSEM Remote API get float.vi"("lpszParam"="AP_FIB_OBJECTIVE_POTENTIAL", "ActiveX Container"=w1619) -> ("vValue"=w1620:sgl)  [unwired: 7 in, 2 out]
            n7570 = local write "FIB Milling Objective (V)"(w1620) -> ()
          }
        }
        n7571 = Select(t=w1603, s=w1602, f=u32 0) -> (s? t:f=w1604:u32)
        n7572 = case shown="True" "FIB time lapse" {
          tunnel: [u32 0 w1870] -> w1616
          tunnel: w1615 -> [_ w1865]
          tunnel: w1570 -> [_ w1864]
          frame False {
          }
          frame True {
            n7573 = Equal To 0?(x=w1865) -> (x = 0?=w1866:bool)
            n7574 = case shown="True" w1866 {
              frame False {
              }
              frame True {
                n7575 = stacked-sequence {
                  frame #0 {
                    n7576 = local read "File Information"() -> (w1876:T31)
                    n7577 = Get Date/Time In Seconds() -> (seconds since 1Jan1904=w1873:timestamp)
                    n7578 = Unbundle By Name(w1876) -> ("File path"=w1875:path)
                    n7579 = Format Date/Time String(time format string (%c)="Y%Y\\M%m\\D%d", seconds (now)=w1873) -> (date/time string=w1878:string)  [unwired: 1 out]
                    n7580 = Build Path(base path=w1875, name or relative path=w1878) -> (appended path=w1874:path)
                    n7581 = Format Date/Time String(time format string (%c)="%y-%m-%d_%H%M%S") -> (date/time string=w1881:string)  [unwired: 1 in, 1 out]
                    n7582 = File/Directory Info(path=w1874) -> (path out=w1884:path, error out=w1886:errorcluster)  [unwired: 1 in, 5 out]
                    n7583 = Concatenate Strings("FIB_" ("string"), w1881, ".png" ("string")) -> (w1887:string)
                    n7584 = Unbundle By Name(w1886) -> ("status"=w1885:bool)
                    n7585 = Build Path(base path=w1874, name or relative path=w1887) -> (appended path=→"FIB file name":path)
                    n7586 = case shown="True" w1885 {
                      tunnel: w1884 -> [_ w1888]
                      frame False {
                      }
                      frame True {
                        n7587 = Create Folder(path (use dialog)=w1888) -> ()  [unwired: 1 in, 4 out]
                      }
                    }
                  }
                  frame #1 {
                    n7588 = local read "Api"() -> (w1889:refnum<k7>)
                    n7589 = local read "FIB HW Config"() -> (w1895:T23)
                    n7590 = local read "FIB HW Config"() -> (w1892:T23)
                    n7591 = Unbundle By Name(w1895) -> ("Beam blank"=w1894:tag)
                    n7592 = Unbundle By Name(w1892) -> ("FIB Ext Scan"=w1890:tag)
                    n7593 = call "FIB beam blank.vi"("ActiveX Container"=w1889, "Beam blanked"=TRUE, "lines"=w1894) -> ()  [unwired: 2 in, 1 out]
                    n7594 = call "FIB ext scan.vi"("Ext on"=TRUE ("data"), "FIB Ext Scan"=w1890) -> ()  [unwired: 9 in, 1 out]
                  }
                  frame #2 {
                    n7595 = local read "Machine Type"() -> (w1896:u8)
                    n7596 = case shown="1" w1896 {
                      frame 0, Default {
                      }
                      frame 1 {
                        w1899 = TRUE ("Close session")
                        n7597 = local read "COM port"() -> (w1901:refnum<visa-resource-name>)
                        n7598 = call "Remcon32 command.vi"("Initialization"=w1899, "SEM command"="edx 1", "COM port in"=w1901) -> ("COM port out"=w1900:refnum<visa-resource-name>)  [unwired: 5 in, 3 out]
                        n7599 = call "FIB mode.vi"("Close session"=w1899, "Iterations"=u32 3, "FIB mode"=T10."FIB", "COM port in"=w1900) -> ()  [unwired: 6 in, 2 out]
                      }
                    }
                  }
                  frame #3 {
                    w1906 = TRUE ("As subVi")
                    n7600 = local read "FIB HW Config"() -> (w1907:T23)
                    n7601 = local read "FIB Options"() -> (w1908:T33)
                    n7602 = local read "FIB Scan Parameters"() -> (w1905:T32)
                    n7603 = local read "Api"() -> (w1903:refnum<k7>)
                    n7604 = call "FIB realtime imaging PXIe-6124.vi"("HW Config"=w1907, "Options"=w1908, "Single scan"=w1906, "Scan Para"=w1905, "As subVi"=w1906, "ActiveX Container"=w1903) -> ()  [unwired: 3 in, 2 out]
                    n7605 = local write "Status message"("FIB imaging" ("Status message")) -> ()
                    n7606 = local write "Image Tabs"(T37."FIB" ("Image Tabs")) -> ()
                  }
                  frame #4 {
                    n7607 = shared-variable ".\\Zeiss Library.lvlib\\FIB Img"() -> (w1911:i16[][])  [unwired: 1 in, 1 out]
                    n7608 = call "16bit Image Normalization.vi"("Transpose"=FALSE, "Input image"=w1911) -> ("Normalized image"=w1914:u8[][])  [unwired: 5 in, 4 out]
                    n7609 = local read "FIB file name"() -> (w1915:path)
                    n7610 = call <vilib>:"Flatten Pixmap.vi"("colors"=u32[] [16777222, 65793, 131586, 197379, 263172, 328965, 394758, 460551, 526344, 592137, 657930, 723723, 789516, 855309, 921102, 986895, 1052688, 1118481, 1184274, 1250067, 1315860, 1381653, 1447446, 1513239, 1579032, 1644825, 1710618, 1776411, 1842204, 1907997, 1973790, 2039583, 2105376, 2171169, 2236962, 2302755, 2368548, 2434341, 2500134, 2565927, 2631720, 2697513, 2763306, 2829099, 2894892, 2960685, 3026478, 3092271, 3158064, 3223857, 3289650, 3355443, 3421236, 3487029, 3552822, 3618615, 3684408, 3750201, 3815994, 3881787, 3947580, 4013373, 4079166, 4144959, 4210752, 4276545, 4342338, 4408131, 4473924, 4539717, 4605510, 4671303, 4737096, 4802889, 4868682, 4934475, 5000268, 5066061, 5131854, 5197647, 5263440, 5329233, 5395026, 5460819, 5526612, 5592405, 5658198, 5723991, 5789784, 5855577, 5921370, 5987163, 6052956, 6118749, 6184542, 6250335, 6316128, 6381921, 6447714, 6513507, 6579300, 6645093, 6710886, 6776679, 6842472, 6908265, 6974058, 7039851, 7105644, 7171437, 7237230, 7303023, 7368816, 7434609, 7500402, 7566195, 7631988, 7697781, 7763574, 7829367, 7895160, 7960953, 8026746, 8092539, 8158332, 8224125, 8289918, 8355711, 8421504, 8487297, 8553090, 8618883, 8684676, 8750469, 8816262, 8882055, 8947848, 9013641, 9079434, 9145227, 9211020, 9276813, 9342606, 9408399, 9474192, 9539985, 9605778, 9671571, 9737364, 9803157, 9868950, 9934743, 10000536, 10066329, 10132122, 10197915, 10263708, 10329501, 10395294, 10461087, 10526880, 10592673, 10658466, 10724259, 10790052, 10855845, 10921638, 10987431, 11053224, 11119017, 11184810, 11250603, 11316396, 11382189, 11447982, 11513775, 11579568, 11645361, 11711154, 11776947, 11842740, 11908533, 11974326, 12040119, 12105912, 12171705, 12237498, 12303291, 12369084, 12434877, 12500670, 12566463, 12632256, 12698049, 12763842, 12829635, 12895428, 12961221, 13027014, 13092807, 13158600, 13224393, 13290186, 13355979, 13421772, 13487565, 13553358, 13619151, 13684944, 13750737, 13816530, 13882323, 13948116, 14013909, 14079702, 14145495, 14211288, 14277081, 14342874, 14408667, 14474460, 14540253, 14606046, 14671839, 14737632, 14803425, 14869218, 14935011, 15000804, 15066597, 15132390, 15198183, 15263976, 15329769, 15395562, 15461355, 15527148, 15592941, 15658734, 15724527, 15790320, 15856113, 15921906, 15987699, 16053492, 16119285, 16185078, 16250871, 16316664, 16382457, 16448250, 16514043, 16579836, 16645629, 16711422, 16448250] ("256 gray scale"), "8-bit pixmap"=w1914) -> ("image data"=w1912:T52)  [unwired: 4 in, 5 out]
                    n7611 = call <vilib>:"Write PNG File.vi"("image data"=w1912, "path to PNG file"=w1915) -> ()  [unwired: 1 in, 9 out]
                  }
                  frame #5 {
